vi "GVHorstSP_ECD.vi"() -> ()   [LabVIEW 2017]
panel:
  out "HorstSP":dbl[](array[numeric])
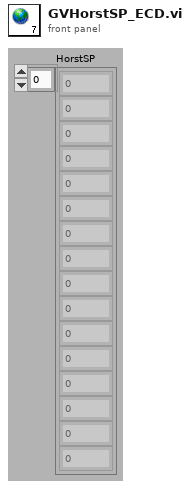
[diagram p1: front panel]
diagram:
